vi "Run.vi"(8 "error in (no error)":errorcluster, 11 "FFT in":refnum<class "FFT.lvclass">) -> (0 "error out":errorcluster, 2 "TimeOut":bool, 3 "FFT out":refnum<class "FFT.lvclass">)   [LabVIEW 2014, in "AnalysisPlugins.lvlib" / "FFT.lvclass"]
uses:
  FFT.lvclass
  FitterBaseClass/FitterBase.lvclass
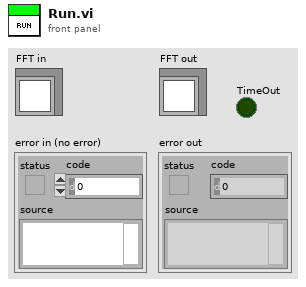
[diagram p1: front panel]
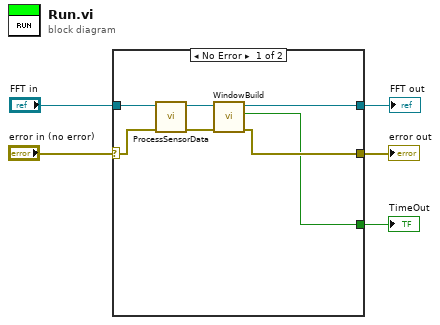
[diagram p0: block diagram]
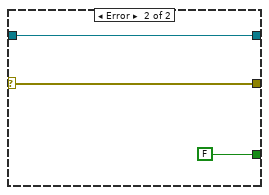
[diagram p2: hidden frame]
diagram:
  n1 = case shown="No Error" "error in (no error)" {
    selector: "error in (no error)" -> [w11 w14]
    tunnel: [w8 w15] -> w3
    tunnel: "FFT in" -> [w12 w15]
    tunnel: [w7 w14] -> w2
    tunnel: [w6 FALSE] -> w1
    frame No Error {
      n2 = call-dynamic "ProcessSensorData.vi"("error in (no error)"=w11, "Class In"=w12) -> ("error out"=w9:errorcluster, "Class Out"=w10:refnum<class "FFT.lvclass">)  [unwired: 8 in]
      n3 = call "WindowBuild.vi"("error in (no error)"=w9, "Fitter in"=w10) -> ("error out"=w7:errorcluster, "Timeout"=w6:bool, "Fitter out"=w8:refnum<class "FFT.lvclass">)  [unwired: 7 in]
    }
    frame Error {
    }
  }
  "error out" <- w2
  "FFT out" <- w3
  "TimeOut" <- w1
